vi "Setup Connection.vi"(0 "NICal5501 in":refnum<class "Cal Standard.lvclass">, 5 "Path Name":string, 11 "error in (no error)":errorcluster) -> (4 "NICal5501 out":refnum<class "Cal Standard.lvclass">, 15 "error out":errorcluster)   [LabVIEW 2023, in "NI Cal-5501 Cal Standard.lvlib" / "Cal Standard.lvclass"]
uses:
  Cal Standard.lvclass
  C:/srd-semi-rfcal-software/AuxTools/STSRFFixtureCharactUtility/Source/Code Modules/Fixture/Instruments/Cal Standard/Cal Standard Base/Cal Standard Base.lvclass
  Properties/Read Product Name.vi
  Instruments/Cal Standard/Cal Standard Base/Cal Standard Base.lvclass
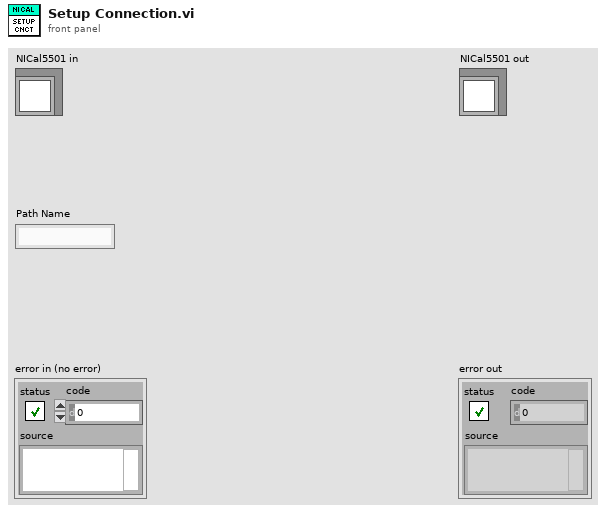
[diagram p1: front panel]
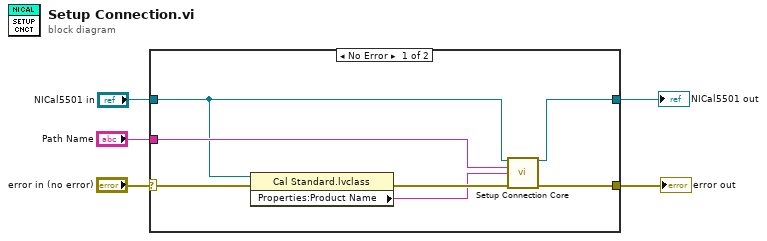
[diagram p0: block diagram]
diagram:
  n1 = case shown="No Error" "error in (no error)" {
    selector: "error in (no error)" -> [w9 w14]
    tunnel: [w11 w14] -> w2
    tunnel: [w10 w13] -> w1
    tunnel: "NICal5501 in" -> [w6 w13]
    tunnel: "Path Name" -> [w12 _]
    frame No Error {
      n2 = property class="Cal Standard.lvclass"(reference=w6, error in=w9) -> (error out=w8:errorcluster, "Properties:Product Name"=w7:string)  [unwired: 1 out]
      n3 = call "Setup Connection Core.vi"("Cal Standard Base in"=w6, "Path Name"=w12, "Product Name"=w7, "error in (no error)"=w8) -> ("Cal Standard Base out"=w10:refnum<class "Cal Standard.lvclass">, "error out"=w11:errorcluster)  [unwired: 10 in]
    }
    frame Error {
    }
  }
  "error out" <- w2
  "NICal5501 out" <- w1
